vi "TGit_LvPlugin_add.vi"() -> ()   [LabVIEW 2018]
uses:
  SHELL32.dll
panel:
  out "Path":string
  # "ツールメニューからこのVIが呼び出されると、呼び出したVIのパスを、エクスプローラで表示します。- Windows専用"
  # "ツールメニューに登録するには、LabVIEWのプログラム保存場所の projectフォルダの下にこのVIを保存するだけです。\nToolMenu Vis path : \"C:\\Program Files\\LabVIEW 2010\\project\\\""
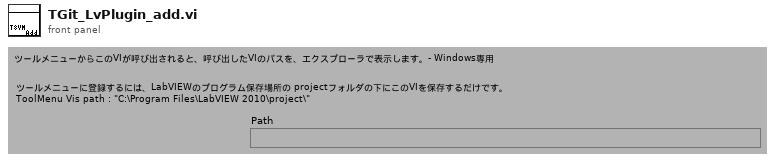
[diagram p1: front panel]
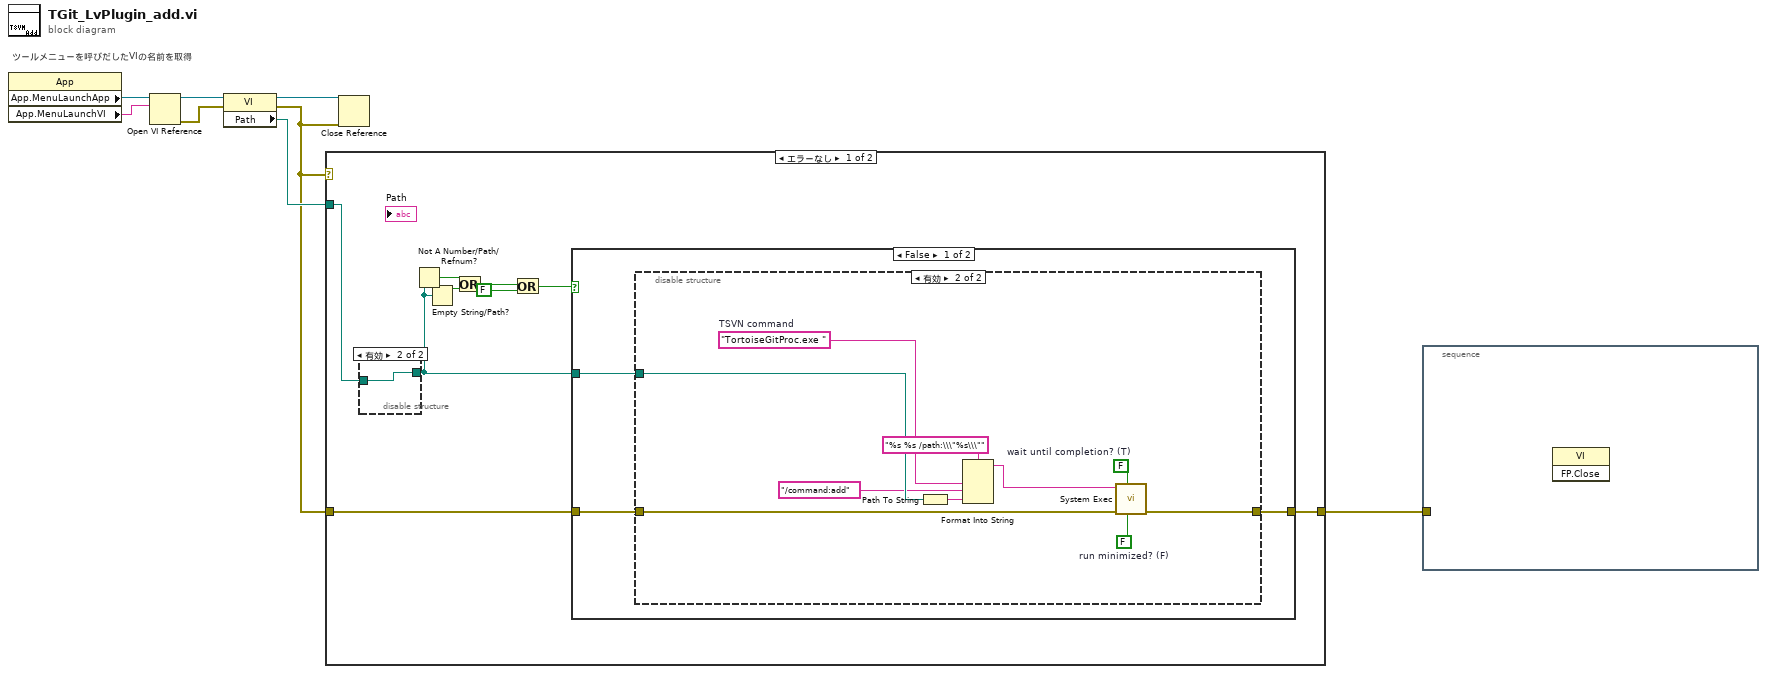
[diagram p0: block diagram]
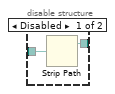
[diagram p2: hidden frame]
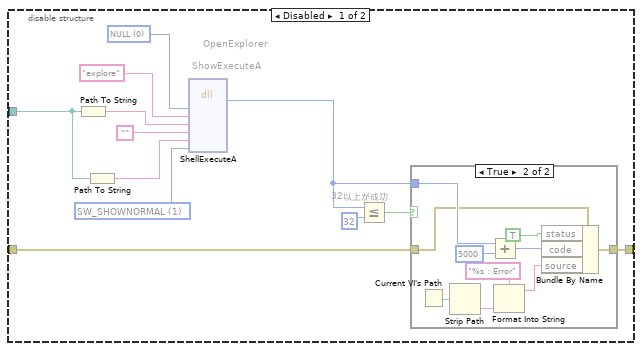
[diagram p3: hidden frame]
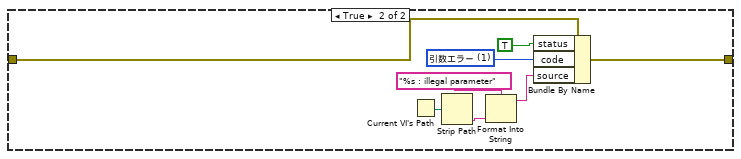
[diagram p5: hidden frame]
diagram:
  # "ツールメニューを呼びだしたVIの名前を取得"
  n1 = property class="App"() -> ("App.MenuLaunchApp"=w7:refnum<vi>, "App.MenuLaunchVI"=w8:string)  [unwired: 2 in, 2 out]
  n2 = Open VI Reference(application reference (local)=w7, vi path=w8) -> (vi reference=w6:refnum<vi>, error out=w5:errorcluster)  [unwired: 4 in]
  n3 = property class="VI"(reference=w6, error in=w5) -> (reference out=w4:refnum<vi>, error out=w2:errorcluster, "Path"=w3:path)
  n4 = case shown="エラーなし" w2 {
    tunnel: w3 -> [w10 _]
    tunnel: w2 -> [w12 w65]
    tunnel: [w11 w65] -> w1
    frame No Error {
      n5 = disable-structure shown="有効" {
        disable-tunnel: w10 -> [w19 w20]
        disable-tunnel: [w18 w20] -> w9
        frame Disabled {
          n6 = Strip Path(path=w19) -> (stripped path=w18:path)  [unwired: 1 out]
        }
        frame Enabled {
        }
      }
      n7 = Not A Number/Path/Refnum?(number/path/refnum=w9) -> (NaN/Path/Refnum?=w17:bool)
      n8 = Empty String/Path?(string/path=w9) -> (empty?=w16:bool)
      n9 = Or(x=w17, y=w16) -> (x .or. y?=w15:bool)
      n10 = Or(x=w15, y=FALSE) -> (x .or. y?=w14:bool)
      n11 = case shown="FALSE" w14 {
        tunnel: [w23 w58] -> w11
        tunnel: w12 -> [w22 w59]
        tunnel: w9 -> [w21 _]
        frame False {
          n12 = disable-structure shown="有効" {
            disable-tunnel: [w32 w53] -> w23
            disable-tunnel: w22 -> [w29 w54]
            disable-tunnel: w21 -> [w27 w50]
            frame Disabled {
              w24 = 1 items=["SW_HIDE", "SW_SHOWNORMAL", "SW_SHOWMINIMIZED"] ("show")
              w28 = 0 items=["NULL"]
              # "OpenExplorer"
              # "ShowExecuteA"
              # "32以上が成功"
              n13 = Path To String(path=w27) -> (string=w35:string)
              n14 = Path To String(path=w27) -> (string=w34:string)
              n15 = dll-call lib="SHELL32.*" fn="ShellExecuteA"("hWndParent"=w28, "lpszOp"="explore", "lpszFile"=w35, "lpszParams"="", "lpszDir"=w34, "fsShowCmd"=w24) -> ("hInstance"=w30:u32)  [unwired: 9 in, 2 out]
              n16 = Less Or Equal?(x=w30, y=u32 32) -> (x <= y?=w31:bool)
              n17 = case shown="TRUE" w31 {
                tunnel: [w36 w46] -> w32
                tunnel: w30 -> [_ w43]
                tunnel: w29 -> [w36 w41]
                frame False {
                }
                frame True {
                  n18 = Current VI's Path() -> (path=w40:path)
                  n19 = Strip Path(path=w40) -> (name=w37:string)  [unwired: 1 out]
                  n20 = Add(x=w43, y=u32 5000) -> (x+y=w44:u32)
                  n21 = Format Into String(format string="%s : Error" ("形式文字列"), w37) -> (resulting string=w38:string)  [unwired: 2 in, 1 out]
                  n22 = Bundle By Name(cluster=w41, "status"=TRUE, "code"=w44, "source"=w38) -> (w46:errorcluster)
                }
              }
            }
            frame Enabled {
              w52 = "TortoiseGitProc.exe "  # TSVN command
              w56 = FALSE  # run minimized? (F)
              w55 = FALSE  # wait until completion? (T)
              n23 = Path To String(path=w50) -> (string=w49:string)
              n24 = Format Into String(format string="%s %s /path:\\\"%s\\\"" ("形式文字列"), w52, "/command:add" ("入力 2"), w49) -> (resulting string=w48:string)  [unwired: 2 in, 1 out]
              n25 = call <vilib>:"System Exec.vi"("run minimized? (F)"=w56, "wait until completion? (T)"=w55, "error in (no error)"=w54, "command line"=w48) -> ("error out"=w53:errorcluster)  [unwired: 4 in, 3 out]
            }
          }
        }
        frame True {
          w64 = 1 items=["エラーなし", "引数エラー", "メモリがいっぱいです", "ゾーン外です", "ファイルの終わりです", "ファイルは既に開かれています", "一般ファイルI/Oエラー", "ファイルが見つかりません", "ファイル権限エラー", "ディスクがいっぱいです", "複製パス", "開かれているファイルが多すぎます", "システム機能が使用不可と設定されています", "リソースファイルが見つかりません", "リソースを追加できません", "リソースが見つかりません", "イメージが見つかりません", "イメージメモリエラー", "ペンが存在しません", "構成タイプが無効です", "構成トークンが見つかりません", "構成パースエラー", "構成メモリエラー", "外部コードフォーマットが無効です", "外部コードオフセットが無効です", "外部コードが存在しません", "ウィンドウがNullです", "ウィンドウの破壊エラー", "メニューがNullです", "印刷が中断されました", "印刷記録が無効です", "印刷のドライバエラー", "印刷中のウィンドウエラー", "印刷中のメモリエラー", "印刷ダイアログエラー", "一般印刷エラー", "デバイスRefnumが無効です", "デバイスが見つかりません", "デバイスのパラメータエラー", "デバイスのユニットエラー", "デバイスが開けません", "デバイスへのコールが中断されました", "一般エラー", "ユーザにより中断されました", "オブジェクトIDが低すぎます", "オブジェクトIDが高すぎます", "オブジェクトはヒープに存在しません", "不明なヒープ", "不明なオブジェクト(無効なDefProc)", "不明なオブジェクト(DefProcが表に存在しない)", "メッセージは範囲外です", "無効な（Nullな）メソッド", "不明なメッセージ", "マネージャコールはサポートされていません", "無効なアドレス", "ネットワーク操作が実行中", "ネットワーク操作がタイムアウトしました", "リソース使用中のため接続できません", "ネットワークの属性がサポートされていません", "ネットワークエラー", "アドレスが使用中です", "システムがメモリ不足です", "接続が中断されました", "接続が拒否されました", "接続していません", "既に接続しています", "接続は終了しました", "初期化エラー(インタアプリケーションマネージャ)", "無効なオカーレンス", "オカーレンスハンドルを待機中", "オカーレンスキューのオーバーフロー", "データログタイプの競合", "未使用です", "タイプを認識できません(インタアプリケーションマネージャ)", "メモリが破損しています", "一時DLLの作成に失敗しました", "CINの古いバージョンです", "ドラッグソケットが見つかりません", "ドロップオブジェクトのロードに失敗しました。", "OLEオブジェクトの登録に失敗しました", "OLEオブジェクトの開放に失敗しました", "形式の指定が一致してません", "不明な形式文字列", "形式の指定が足りません", "形式の指定が多すぎます", "スキャンに失敗しました", "新しいCINのバージョン", "バリアントへの変換エラー", "ランタイムのメニューエラー", "パスワードが変更されています", "バリアント属性は見つかりませんでした。", "不適合なバリアントデータタイプ", "イベントデータは利用できません", "イベント記憶領域は存在しません", "オカーレンスが見つかりません", "イベント待ち行列が作成されていません", "イベント情報は利用できません", "渡されたRefnumNULLです", "クラスGUIDの回収エラー", "共通クラスGUIDの回収エラー", "タイプライブラリGUIDの回収エラー", "不良アプリケーションmagicバイト", "特定のドライバは論理名に関連付けられた特定のドライバとは異なります。", "クラスドライバに対してセッションが開かれていません。", "Maxエラー", "MAX - 構成オブジェクトのエラー", "MAX - 構成のロードエラー", "MAX - グループはサポートされていません。"]
          n26 = Current VI's Path() -> (path=w62:path)
          n27 = Strip Path(path=w62) -> (name=w57:string)  [unwired: 1 out]
          n28 = Format Into String(format string="%s : illegal parameter" ("形式文字列"), w57) -> (resulting string=w60:string)  [unwired: 2 in, 1 out]
          n29 = Bundle By Name(cluster=w59, "status"=TRUE, "code"=w64, "source"=w60) -> (w58:errorcluster)
        }
      }
    }
    frame Error {
    }
  }
  n30 = Close Reference(reference=w4, error in (no error)=w2) -> ()  [unwired: 1 out]
  n31 = stacked-sequence {
    tunnel: w1 -> [_]
    frame #0 {
      n32 = invoke class="VI" method="FP.Close"() -> ()  [unwired: 3 in, 3 out]
    }
  }
